vi "6733_Write_daqmx_87Sr.vi"(0 "Arbitrary Waveform\nArray of Channels":T1(array[cluster])=[[{"AC Frequency (kHz)"=40.0, " Initial AC Ampl. (p-p/2)"=0.0, "Final AC Ampl."=0.0, "Initial DC Value"=1.2, "Final DC Value"=0.6, "Constant"=80.29, "Gamma AC"=1.0, "String"="Channel 0 A", "Gamma DC"=1.0}, {"AC Frequency (kHz)"=40.0, " Initial AC Ampl. (p-p/2)"=0.0, "Final AC Ampl."=0.0, "Initial DC Value"=0.6, "Final DC Value"=0.2, "Constant"=80.29, "Gamma AC"=1.0, "String"="Channel 0 B", "Gamma DC"=1.0}, {"AC Frequency (kHz)"=40.0, " Initial AC Ampl. (p-p/2)"=0.0, "Final AC Ampl."=0.0, "Initial DC Value"=0.2, "Final DC Value"=0.075, "Constant"=80.29, "Gamma AC"=1.0, "String"="Channel 0 C", "Gamma DC"=1.0}, {"AC Frequency (kHz)"=0.0, " Initial AC Ampl. (p-p/2)"=0.0, "Final AC Ampl."=0.0, "Initial DC Value"=0.0, "Final DC Value"=1.8, "Constant"=84.5, "Gamma AC"=0.0, "String"="Channel 0 D", "Gamma DC"=1.0}, {"AC Frequency (kHz)"=0.0, " Initial AC Ampl. (p-p/2)"=0.0, "Final AC Ampl."=0.0, "Initial DC Value"=0.0, "Final DC Value"=0.0, "Constant"=81.22, "Gamma AC"=0.0, "String"="Channel 0 E", "Gamma DC"=1.0}, {"AC Frequency (kHz)"=0.0, " Initial AC Ampl. (p-p/2)"=0.0, "Final AC Ampl."=0.0, "Initial DC Value"=0.0, "Final DC Value"=0.0, "Constant"=86.0, "Gamma AC"=0.0, "String"="Channel 0 F", "Gamma DC"=1.0}], [{"AC Frequency (kHz)"=10.0, " Initial AC Ampl. (p-p/2)"=5.0, "Final AC Ampl."=0.0, "Initial DC Value"=1.0, "Final DC Value"=0.3, "Constant"=0.0, "Gamma AC"=1.0, "String"="Channel 1 A", "Gamma DC"=1.0}, {"AC Frequency (kHz)"=10.0, " Initial AC Ampl. (p-p/2)"=5.0, "Final AC Ampl."=0.0, "Initial DC Value"=0.3, "Final DC Value"=-0.8, "Constant"=0.0, "Gamma AC"=1.0, "String"="Channel 1 B", "Gamma DC"=1.0}, {"AC Frequency (kHz)"=10.0, " Initial AC Ampl. (p-p/2)"=0.0, "Final AC Ampl."=0.0, "Initial DC Value"=-0.8, "Final DC Value"=-0.8, "Constant"=0.0, "Gamma AC"=1.0, "String"="Channel 1 C", "Gamma DC"=1.0}, {"AC Frequency (kHz)"=0.0, " Initial AC Ampl. (p-p/2)"=0.0, "Final AC Ampl."=0.0, "Initial DC Value"=-1.0, "Final DC Value"=-1.0, "Constant"=0.0, "Gamma AC"=0.0, "String"="Channel 1 D", "Gamma DC"=1.0}, {"AC Frequency (kHz)"=0.0, " Initial AC Ampl. (p-p/2)"=0.0, "Final AC Ampl."=0.0, "Initial DC Value"=-1.0, "Final DC Value"=-1.0, "Constant"=0.0, "Gamma AC"=0.0, "String"="Channel 1E", "Gamma DC"=1.0}, {"AC Frequency (kHz)"=0.0, " Initial AC Ampl. (p-p/2)"=0.0, "Final AC Ampl."=0.0, "Initial DC Value"=-1.0, "Final DC Value"=-1.0, "Constant"=0.0, "Gamma AC"=0.0, "String"="", "Gamma DC"=1.0}], [{"AC Frequency (kHz)"=10.0, " Initial AC Ampl. (p-p/2)"=0.0, "Final AC Ampl."=0.0, "Initial DC Value"=0.01, "Final DC Value"=0.04, "Constant"=0.0, "Gamma AC"=1.0, "String"="Channel 2 A", "Gamma DC"=1.0}, {"AC Frequency (kHz)"=10.0, " Initial AC Ampl. (p-p/2)"=0.0, "Final AC Ampl."=0.0, "Initial DC Value"=0.04, "Final DC Value"=0.1, "Constant"=0.0, "Gamma AC"=1.0, "String"="Channel 2 B", "Gamma DC"=1.0}, {"AC Frequency (kHz)"=10.0, " Initial AC Ampl. (p-p/2)"=0.0, "Final AC Ampl."=0.0, "Initial DC Value"=0.1, "Final DC Value"=0.1, "Constant"=0.0, "Gamma AC"=1.0, "String"="Channel 2 C", "Gamma DC"=1.0}, {"AC Frequency (kHz)"=0.0, " Initial AC Ampl. (p-p/2)"=0.0, "Final AC Ampl."=0.0, "Initial DC Value"=0.1, "Final DC Value"=0.1, "Constant"=0.0, "Gamma AC"=0.0, "String"="Channel 2 D", "Gamma DC"=1.0}, {"AC Frequency (kHz)"=0.0, " Initial AC Ampl. (p-p/2)"=0.0, "Final AC Ampl."=0.0, "Initial DC Value"=0.1, "Final DC Value"=0.1, "Constant"=0.0, "Gamma AC"=0.0, "String"="", "Gamma DC"=1.0}, {"AC Frequency (kHz)"=0.0, " Initial AC Ampl. (p-p/2)"=0.0, "Final AC Ampl."=0.0, "Initial DC Value"=0.1, "Final DC Value"=0.1, "Constant"=0.0, "Gamma AC"=0.0, "String"="", "Gamma DC"=1.0}], [{"AC Frequency (kHz)"=10.0, " Initial AC Ampl. (p-p/2)"=0.0, "Final AC Ampl."=0.0, "Initial DC Value"=10.0, "Final DC Value"=10.0, "Constant"=199.25, "Gamma AC"=1.0, "String"="Channel 3 A", "Gamma DC"=1.0}, {"AC Frequency (kHz)"=10.0, " Initial AC Ampl. (p-p/2)"=0.0, "Final AC Ampl."=0.0, "Initial DC Value"=10.0, "Final DC Value"=0.8, "Constant"=199.25, "Gamma AC"=1.0, "String"="Channel 3 B", "Gamma DC"=1.0}, {"AC Frequency (kHz)"=10.0, " Initial AC Ampl. (p-p/2)"=0.0, "Final AC Ampl."=0.0, "Initial DC Value"=1.0, "Final DC Value"=0.5, "Constant"=199.25, "Gamma AC"=1.0, "String"="Channel 3 C", "Gamma DC"=1.0}, {"AC Frequency (kHz)"=0.0, " Initial AC Ampl. (p-p/2)"=0.0, "Final AC Ampl."=0.0, "Initial DC Value"=1.0, "Final DC Value"=1.0, "Constant"=199.25, "Gamma AC"=0.0, "String"="Channel 3 D", "Gamma DC"=1.0}, {"AC Frequency (kHz)"=0.0, " Initial AC Ampl. (p-p/2)"=0.0, "Final AC Ampl."=0.0, "Initial DC Value"=0.6, "Final DC Value"=0.6, "Constant"=199.2, "Gamma AC"=0.0, "String"="", "Gamma DC"=1.0}, {"AC Frequency (kHz)"=0.0, " Initial AC Ampl. (p-p/2)"=0.0, "Final AC Ampl."=0.0, "Initial DC Value"=0.6, "Final DC Value"=0.6, "Constant"=199.2, "Gamma AC"=0.0, "String"="", "Gamma DC"=1.0}], [{"AC Frequency (kHz)"=10.0, " Initial AC Ampl. (p-p/2)"=0.0, "Final AC Ampl."=0.0, "Initial DC Value"=-1.2, "Final DC Value"=-0.6, "Constant"=221.72, "Gamma AC"=1.0, "String"="Channel 4 A", "Gamma DC"=1.0}, {"AC Frequency (kHz)"=10.0, " Initial AC Ampl. (p-p/2)"=0.0, "Final AC Ampl."=0.0, "Initial DC Value"=-0.6, "Final DC Value"=-0.2, "Constant"=221.72, "Gamma AC"=1.0, "String"="Channel 4 B", "Gamma DC"=1.0}, {"AC Frequency (kHz)"=10.0, " Initial AC Ampl. (p-p/2)"=0.0, "Final AC Ampl."=0.0, "Initial DC Value"=-0.2, "Final DC Value"=-0.075, "Constant"=221.72, "Gamma AC"=1.0, "String"="Channel 4 C", "Gamma DC"=1.0}, {"AC Frequency (kHz)"=0.0, " Initial AC Ampl. (p-p/2)"=0.0, "Final AC Ampl."=0.0, "Initial DC Value"=0.0, "Final DC Value"=0.0, "Constant"=221.69, "Gamma AC"=0.0, "String"="Channel 4 D", "Gamma DC"=1.0}, {"AC Frequency (kHz)"=0.0, " Initial AC Ampl. (p-p/2)"=0.0, "Final AC Ampl."=0.0, "Initial DC Value"=0.0, "Final DC Value"=0.0, "Constant"=221.85, "Gamma AC"=0.0, "String"="", "Gamma DC"=1.0}, {"AC Frequency (kHz)"=0.0, " Initial AC Ampl. (p-p/2)"=0.0, "Final AC Ampl."=0.0, "Initial DC Value"=0.0, "Final DC Value"=0.0, "Constant"=221.85, "Gamma AC"=0.0, "String"="", "Gamma DC"=1.0}], [{"AC Frequency (kHz)"=10.0, " Initial AC Ampl. (p-p/2)"=0.0, "Final AC Ampl."=0.0, "Initial DC Value"=10.0, "Final DC Value"=10.0, "Constant"=0.0, "Gamma AC"=1.0, "String"="Channel 5 A", "Gamma DC"=1.0}, {"AC Frequency (kHz)"=10.0, " Initial AC Ampl. (p-p/2)"=0.0, "Final AC Ampl."=0.0, "Initial DC Value"=10.0, "Final DC Value"=0.8, "Constant"=0.0, "Gamma AC"=1.0, "String"="Channel 5 B", "Gamma DC"=1.0}, {"AC Frequency (kHz)"=10.0, " Initial AC Ampl. (p-p/2)"=0.0, "Final AC Ampl."=0.0, "Initial DC Value"=1.0, "Final DC Value"=0.5, "Constant"=0.0, "Gamma AC"=1.0, "String"="Channel 5 C", "Gamma DC"=1.0}, {"AC Frequency (kHz)"=0.0, " Initial AC Ampl. (p-p/2)"=0.0, "Final AC Ampl."=0.0, "Initial DC Value"=0.47, "Final DC Value"=0.47, "Constant"=0.0, "Gamma AC"=0.0, "String"="Channel 5 D", "Gamma DC"=1.0}, {"AC Frequency (kHz)"=0.0, " Initial AC Ampl. (p-p/2)"=0.0, "Final AC Ampl."=0.0, "Initial DC Value"=10.0, "Final DC Value"=10.0, "Constant"=0.0, "Gamma AC"=0.0, "String"="", "Gamma DC"=1.0}, {"AC Frequency (kHz)"=0.0, " Initial AC Ampl. (p-p/2)"=0.0, "Final AC Ampl."=0.0, "Initial DC Value"=10.0, "Final DC Value"=10.0, "Constant"=0.0, "Gamma AC"=0.0, "String"="", "Gamma DC"=1.0}], [{"AC Frequency (kHz)"=10.0, " Initial AC Ampl. (p-p/2)"=0.0, "Final AC Ampl."=0.0, "Initial DC Value"=1.0, "Final DC Value"=0.0, "Constant"=0.0, "Gamma AC"=1.0, "String"="Channel 6 A", "Gamma DC"=1.0}, {"AC Frequency (kHz)"=10.0, " Initial AC Ampl. (p-p/2)"=0.0, "Final AC Ampl."=0.0, "Initial DC Value"=0.0, "Final DC Value"=-0.7, "Constant"=0.0, "Gamma AC"=1.0, "String"="Channel 6 B", "Gamma DC"=1.0}, {"AC Frequency (kHz)"=10.0, " Initial AC Ampl. (p-p/2)"=0.0, "Final AC Ampl."=0.0, "Initial DC Value"=-0.8, "Final DC Value"=-0.8, "Constant"=0.0, "Gamma AC"=1.0, "String"="Channel 6 C", "Gamma DC"=1.0}, {"AC Frequency (kHz)"=0.0, " Initial AC Ampl. (p-p/2)"=0.0, "Final AC Ampl."=0.0, "Initial DC Value"=-1.0, "Final DC Value"=-1.0, "Constant"=0.0, "Gamma AC"=0.0, "String"="Channel 6 D", "Gamma DC"=1.0}, {"AC Frequency (kHz)"=0.0, " Initial AC Ampl. (p-p/2)"=0.0, "Final AC Ampl."=0.0, "Initial DC Value"=1.0, "Final DC Value"=1.0, "Constant"=0.0, "Gamma AC"=0.0, "String"="", "Gamma DC"=1.0}, {"AC Frequency (kHz)"=0.0, " Initial AC Ampl. (p-p/2)"=0.0, "Final AC Ampl."=0.0, "Initial DC Value"=1.0, "Final DC Value"=1.0, "Constant"=0.0, "Gamma AC"=0.0, "String"="", "Gamma DC"=1.0}], [{"AC Frequency (kHz)"=10.0, " Initial AC Ampl. (p-p/2)"=0.0, "Final AC Ampl."=0.0, "Initial DC Value"=1.0, "Final DC Value"=1.0, "Constant"=0.0, "Gamma AC"=1.0, "String"="Channel 7 A", "Gamma DC"=1.0}, {"AC Frequency (kHz)"=10.0, " Initial AC Ampl. (p-p/2)"=0.0, "Final AC Ampl."=0.0, "Initial DC Value"=1.0, "Final DC Value"=1.0, "Constant"=0.0, "Gamma AC"=1.0, "String"="Channel 7 B", "Gamma DC"=1.0}, {"AC Frequency (kHz)"=10.0, " Initial AC Ampl. (p-p/2)"=0.0, "Final AC Ampl."=0.0, "Initial DC Value"=1.0, "Final DC Value"=1.0, "Constant"=0.0, "Gamma AC"=1.0, "String"="Channel 7 C", "Gamma DC"=1.0}, {"AC Frequency (kHz)"=0.0, " Initial AC Ampl. (p-p/2)"=0.0, "Final AC Ampl."=0.0, "Initial DC Value"=1.0, "Final DC Value"=1.0, "Constant"=0.0, "Gamma AC"=0.0, "String"="Channel 7 D", "Gamma DC"=1.0}, {"AC Frequency (kHz)"=0.0, " Initial AC Ampl. (p-p/2)"=0.0, "Final AC Ampl."=0.0, "Initial DC Value"=1.0, "Final DC Value"=1.0, "Constant"=0.0, "Gamma AC"=0.0, "String"="", "Gamma DC"=1.0}, {"AC Frequency (kHz)"=0.0, " Initial AC Ampl. (p-p/2)"=0.0, "Final AC Ampl."=0.0, "Initial DC Value"=2.46, "Final DC Value"=2.46, "Constant"=199.2, "Gamma AC"=0.0, "String"="", "Gamma DC"=1.0}]] {"Gamma DC" format="%.2f"; "Gamma AC" format="%.2f"; "Constant" min=0.0 max=1250.0 format="%.2f"; "Final DC Value" format="%.3f"; "Initial DC Value" format="%.3f"; "Final AC Ampl." format="%.3f"; "Initial AC Ampl. (p-p/2)" format="%.3f"; "AC Frequency (kHz)" format="%.2f"}, 3 "Unit Conversions":u16[](array[ring])=[0, 2, 2, 3, 4, 3, 2, 2] items=["Freq (MHz) to Voltage 87Sr Trap", "87Sr Trap Dither Amplitude", "B-field to Voltage", "Power Control V for 689 nm (%)", "Freq (MHz) to Voltage 87Sr Stir", "Current (A) to Voltage Fet switch X trim", "87Sr Stir Dither Amplitude"], 4 "Interval Lengths (ms)":dbl[](array[numeric])=[200.0, 200.0, 100.0, 150.0, 1.0, 50.0] format="%.3f", 5 "Channel Controls":bool[](array[boolean])=[TRUE, TRUE, TRUE, TRUE, TRUE, TRUE, TRUE, TRUE], 6 "ON or OFF?":bool[](array[boolean])=[TRUE, TRUE, TRUE, TRUE, TRUE, TRUE], 7 "Hold Final Value of Array?":bool=TRUE, 9 "error in":errorcluster, 12 "Dither Control":u16(ring)=1 items=["Disable Dither", "Enable Dither"]) -> (8 "Voltage\nArrays":dbl[][](graph), 10 "= Total Waveform\nTime (ms)":dbl=651.0 format="%.3f", 11 "Sampling\nRate":dbl=3135.593220338983 format="%.2f", 14 "87Sr Trap V":dbl=2.8350019729729716, 15 "error out":errorcluster)   [LabVIEW 2013]
uses:
  <vilib>/Utility/error.llb/DialogType.ctl
  <vilib>/DAQmx/write.llb/DAQmx Write (Analog 1D Wfm NChan NSamp).vi
  <vilib>/DAQmx/configure/timing.llb/DAQmx Timing (Sample Clock).vi
  <vilib>/DAQmx/create/channels.llb/DAQmx Create Channel (CO-Pulse Generation-Frequency).vi
  <vilib>/DAQmx/configure/timing.llb/DAQmx Timing (Implicit).vi
  <vilib>/DAQmx/configure/trigger.llb/DAQmx Start Trigger (Digital Edge).vi
  Instance          13 29Saved   6733_Write_daqmx_87Sr .vi
  <vilib>/DAQmx/miscellaneous.llb/DAQmx Fill In Error Info.vi
  <resource>/objmgr/daqmx.rc
panel:
  in  "Case Constant\n(See Context Help) 3":bool=TRUE
  in  "Dither Control":u16
  in  "Dither Control":u16
  in  "Case Constant\n(See Context Help) 2":bool
  in  "Dither Control":u16
  in  "Case Constant\n(See Context Help)":bool
  in  "Dither Control":u16
  out "87Sr Stir V":dbl=5.786668445945946
  out "wvfrm size":i32=2040
  out "signal out":waveform(dbl)[](graph)=[{"t0"=timestamp(0 s since 1904-01-01), "dt"=0.00031891891891891894, "Y"=array[2040 elements]}, {"t0"=timestamp(0 s since 1904-01-01), "dt"=0.00031891891891891894, "Y"=array[2040 elements]}, {"t0"=timestamp(0 s since 1904-01-01), "dt"=0.00031891891891891894, "Y"=array[2040 elements]}, {"t0"=timestamp(0 s since 1904-01-01), "dt"=0.00031891891891891894, "Y"=array[2040 elements]}, {"t0"=timestamp(0 s since 1904-01-01), "dt"=0.00031891891891891894, "Y"=array[2040 elements]}, {"t0"=timestamp(0 s since 1904-01-01), "dt"=0.00031891891891891894, "Y"=array[2040 elements]}, {"t0"=timestamp(0 s since 1904-01-01), "dt"=0.00031891891891891894, "Y"=array[2040 elements]}, {"t0"=timestamp(0 s since 1904-01-01), "dt"=0.00031891891891891894, "Y"=array[2040 elements]}]
  out "87Sr 6733 counter task out":refnum<k21>="87Sr 6733 Counter Output"
  out "87Sr 6733 adiabatic loading task out":refnum<k21>="87Sr Red Waveform"
  out "6733 Status":string="PCI-6733 OK"
  out "total points\nper channel":dbl=2041.0 format="%.2f"
  out "Points per Segment":dbl[](array[numeric])=[627.0, 627.0, 313.0, 470.0, 3.0] format="%.2f"
  # "Controls"
  # "Warning! Constant for interval A does not set all intervals for 86 Sr frequency"
  # "Don't change"
  # "Note: B-field to Voltage\nConversion not yet\nimplemented.  Must \ninsert appropriate\nformulae."
  # "Interval A"
  # "Interval B"
  # "Interval C"
  # "Interval D"
  # "Interval E"
  # "Output"
  # "Must use all channels"
  # "CH 0"
  # "CH 1"
  # "CH 2"
  # "CH 3"
  # "CH 4"
  # "CH 5"
  # "CH 6"
  # "CH 7"
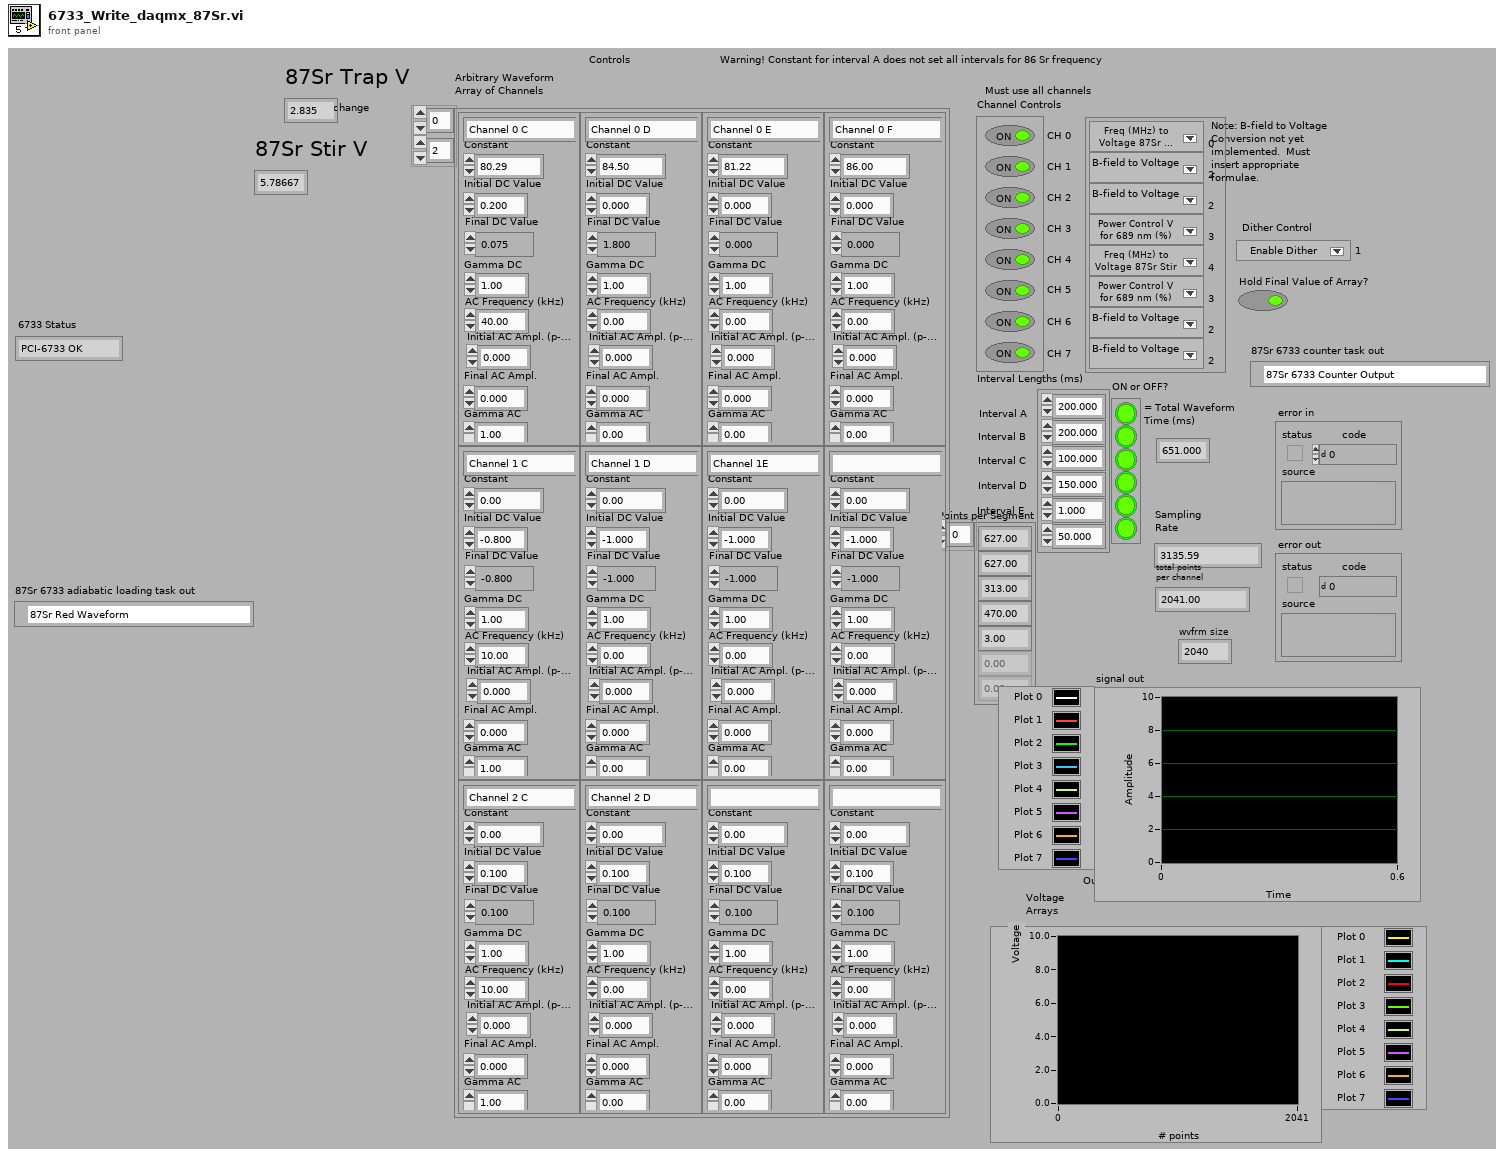
[diagram p1: front panel]
types:
  T1 = cluster{"AC Frequency (kHz)":dbl, " Initial AC Ampl. (p-p/2)":dbl, "Final AC Ampl.":dbl, "Initial DC Value":dbl, "Final DC Value":dbl, "Constant":dbl, "Gamma AC":dbl, "String":string, "Gamma DC":dbl}[][]
  T2 = cluster{"AC Frequency (kHz)":dbl, " Initial AC Ampl. (p-p/2)":dbl, "Final AC Ampl.":dbl, "Initial DC Value":dbl, "Final DC Value":dbl, "Constant":dbl, "Gamma AC":dbl, "String":string, "Gamma DC":dbl}
  T3 = typedef "DialogType.ctl" = u16
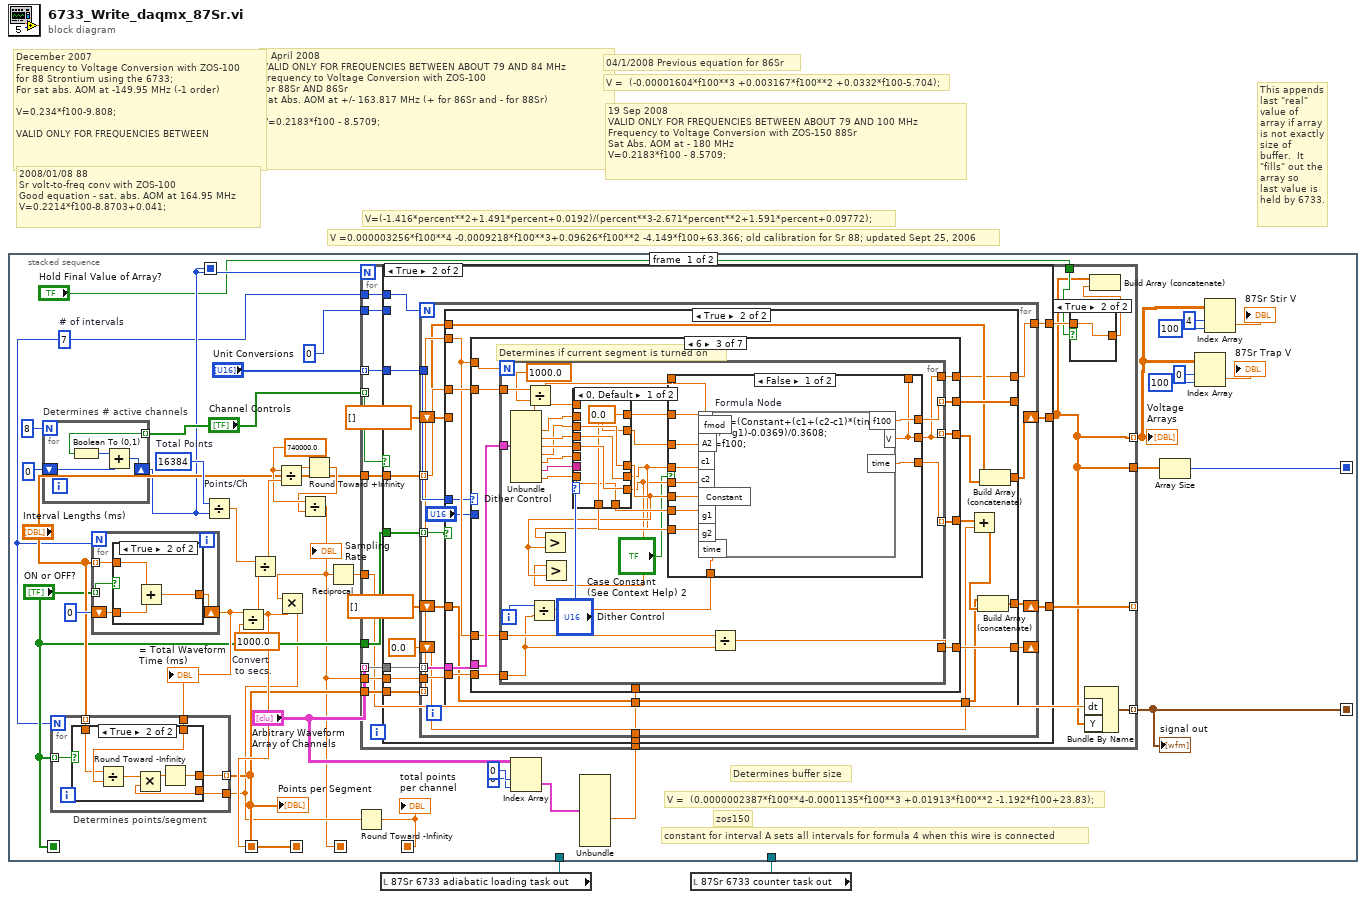
[diagram p0: block diagram]
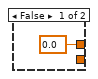
[diagram p2: hidden frame]
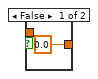
[diagram p4: hidden frame]
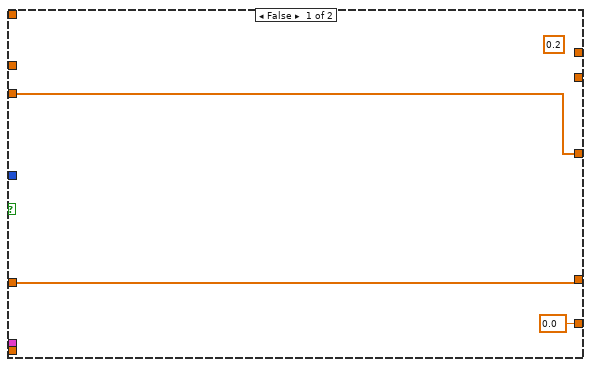
[diagram p6: hidden frame]
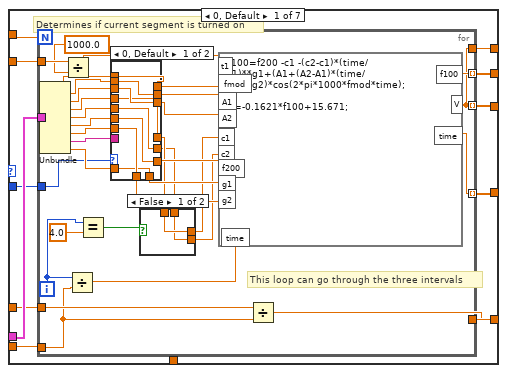
[diagram p7: hidden frame]
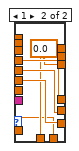
[diagram p9: hidden frame]
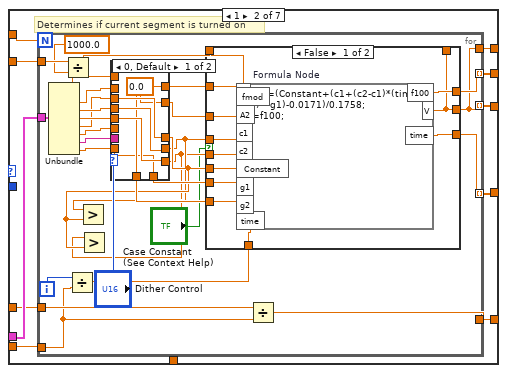
[diagram p10: hidden frame]
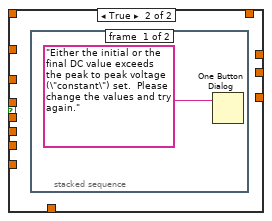
[diagram p11: hidden frame]
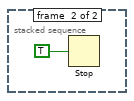
[diagram p12: hidden frame]
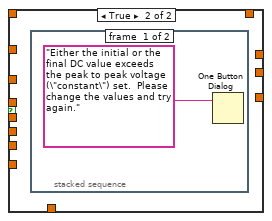
[diagram p14: hidden frame]
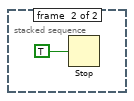
[diagram p15: hidden frame]
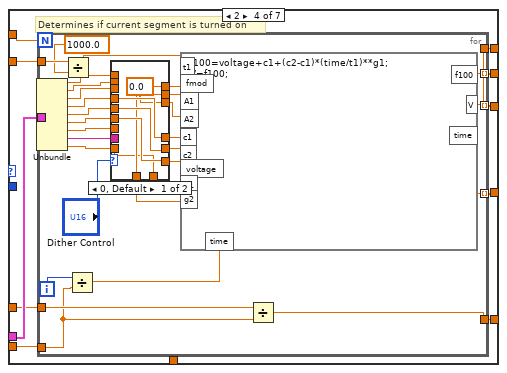
[diagram p17: hidden frame]
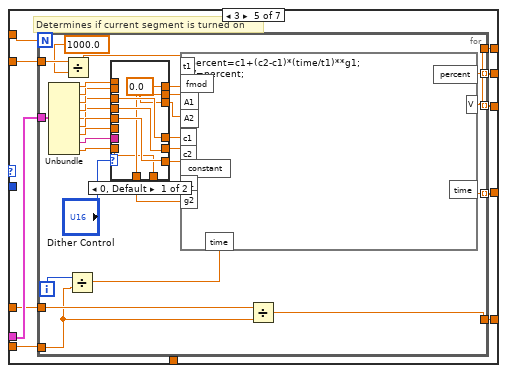
[diagram p19: hidden frame]
diagram:
  # "19 Sep 2008\nVALID ONLY FOR FREQUENCIES BETWEEN ABOUT 79 AND 100 MHz\nFrequency to Voltage Conversion with ZOS-150 88Sr\nSat Abs. AOM at - 180 MHz\nV=0.2183*f100 - 8.5709;"
  # "7 April 2008\nVALID ONLY FOR FREQUENCIES BETWEEN ABOUT 79 AND 84 MHz\nFrequency to Voltage Conversion with ZOS-100\nfor 88Sr AND 86Sr\nSat Abs. AOM at +/- 163.817 MHz (+ for 86Sr and - for 88Sr)\n\nV=0.2183*f100 - 8.5709;"
  # "04/1/2008 Previous equation for 86Sr"
  # "V =  (-0.00001604*f100**3 +0.003167*f100**2 +0.0332*f100-5.704);"
  # "December 2007\nFrequency to Voltage Conversion with ZOS-100\nfor 88 Strontium using the 6733; \nFor sat abs. AOM at -149.95 MHz (-1 order)\n\nV=0.234*f100-9.808;\n\nVALID ONLY FOR FREQUENCIES BETWEEN"
  # "2008/01/08 88\nSr volt-to-freq conv with ZOS-100\nGood equation - sat. abs. AOM at 164.95 MHz\nV=0.2214*f100-8.8703+0.041;"
  # "This appends\nlast \"real\"\nvalue of\narray if array \nis not exactly\nsize of \nbuffer.  It\n\"fills\" out the\narray so \nlast value is\nheld by 6733."
  # "V =0.000003256*f100**4 -0.0009218*f100**3+0.09626*f100**2 -4.149*f100+63.366; old calibration for Sr 88; updated Sept 25, 2006"
  # "V=(-1.416*percent**2+1.491*percent+0.0192)/(percent**3-2.671*percent**2+1.591*percent+0.09772);"
  n1 = local read "87Sr 6733 adiabatic loading task out"() -> (w2:refnum<k21>)
  n2 = local read "87Sr 6733 counter task out"() -> (w1:refnum<k21>)
  n3 = stacked-sequence {
    seq-local: [w13 _] -> [_ w543]
    seq-local: [w26 _] -> [_ _]
    seq-local: ["ON or OFF?" _] -> [_ _]
    seq-local: [w23 _] -> [_ _]
    seq-local: [w28 _] -> [_ _]
    seq-local: [w17 _] -> [_ w590]
    seq-local: [w14 _] -> [_ w542]
    seq-local: [w11 _] -> [_ w541]
    tunnel: w2 -> [_ w581]
    tunnel: w1 -> [_ w580]
    frame #0 {
      w32 = 740000.0 ("x")
      w10 = 7  # # of intervals
      w42 = 16384  # Total Points
      # "zos150"
      # "Determines buffer size"
      # "constant for interval A sets all intervals for formula 4 when this wire is connected"
      # "V =  (0.0000002387*f100**4-0.0001135*f100**3 +0.01913*f100**2 -1.192*f100+23.83);"
      n4 = for "Determines # active channels" {
        N: 8 -> [_]
        tunnel: "Channel Controls" -> [w66] mode=indexing
        shift-right: [w63] -> w17
        shift-left: 0 -> [w64]
        n5 = Boolean To (0,1)(Boolean=w66) -> (0, 1=w65:i16)
        n6 = Add(x=w65, y=w64) -> (x+y=w63:i32)
      }
      n7 = for {
        N: w10 -> [_]
        tunnel: "Interval Lengths (ms)" -> [w56] mode=indexing
        tunnel: "ON or OFF?" -> [w58] mode=indexing
        shift-right: [w55] -> w29
        shift-left: 0 -> [w57]
        n8 = case shown="True" w58 {
          tunnel: w57 -> [w59 w62]
          tunnel: w56 -> [_ w61]
          tunnel: [w59 w60] -> w55
          frame False {
          }
          frame True {
            n9 = Add(x=w61, y=w62) -> (x+y=w60:dbl)
          }
        }
      }
      "= Total Waveform\nTime (ms)" <- w29
      n10 = Divide "Points/Ch"(x=w42, y=w17) -> (x/y=w27:dbl)
      n11 = Divide "Convert\n to secs."(x=w29, y=1000.0) -> (x/y=w28:dbl)
      n12 = Divide(x=w27, y=w28) -> (x/y=w34:dbl)
      n13 = Divide(x=w32, y=w34) -> (x/y=w33:dbl)
      n14 = Round Toward +Infinity(x=w33) -> (ceil(x): smallest int >= x=w31:dbl)
      n15 = Divide(x=w32, y=w31) -> (x/y=w13:dbl)
      "Sampling\nRate" <- w13
      n16 = Multiply(x=w13, y=w28) -> (x*y=w24:dbl)
      n17 = for "Determines points/segment" {
        N: w10 -> [_]
        tunnel: "ON or OFF?" -> [w47] mode=indexing
        tunnel: "Interval Lengths (ms)" -> [w46] mode=indexing
        tunnel: w29 -> [w45]
        tunnel: [w44] -> w26 mode=indexing
        tunnel: w24 -> [w43]
        n18 = case shown="True" w47 {
          tunnel: w46 -> [_ w53]
          tunnel: w45 -> [_ w54]
          tunnel: [0.0 w50] -> w44
          tunnel: w43 -> [_ w51]
          frame False {
          }
          frame True {
            n19 = Divide(x=w53, y=w54) -> (x/y=w52:dbl)
            n20 = Multiply(x=w52, y=w51) -> (x*y=w49:dbl)
            n21 = Round Toward -Infinity(1:w49) -> (0:w50:dbl)
          }
        }
      }
      "Points per Segment" <- w26
      n22 = Reciprocal(x=w13) -> (1/x=w15:dbl)
      n23 = Round Toward -Infinity(1:w24) -> (0:w23:dbl)
      "total points\nper channel" <- w23
      n24 = Index Array(array="Arbitrary Waveform\nArray of Channels", index (row)=0, index (col)=0 ("disabled index (col)")) -> (element=w19:T2)
      n25 = Unbundle(w19) -> ("Constant"=w18:dbl)  [unwired: 8 out]
      n26 = for {
        N: w17 -> [_]
        tunnel: "Channel Controls" -> [w83] mode=indexing
        tunnel: 0 -> [w82]
        tunnel: "Unit Conversions" -> [w80] mode=indexing
        tunnel: "Arbitrary Waveform\nArray of Channels" -> [w81] mode=indexing
        tunnel: w26 -> [w79]
        tunnel: w13 -> [w70]
        tunnel: "Interval Lengths (ms)" -> [w78]
        tunnel: "ON or OFF?" -> [w77]
        tunnel: [w76] -> _ mode=indexing
        tunnel: [w67] -> w3 mode=indexing
        tunnel: w18 -> [w75]
        tunnel: "Hold Final Value of Array?" -> [w72]
        tunnel: [w71] -> w14 mode=indexing
        tunnel: w15 -> [w69]
        tunnel: [w67] -> w12
        tunnel: w10 -> [w68]
        n27 = case shown="True" w83 {
          tunnel: w82 -> [_ _]
          tunnel: w81 -> [_ w99]
          tunnel: w80 -> [_ w98]
          tunnel: w79 -> [_ w97]
          tunnel: w70 -> [_ w96]
          tunnel: w78 -> [_ w95]
          tunnel: w77 -> [_ w94]
          tunnel: [_ w92] -> w76
          tunnel: [_ w87] -> w67
          tunnel: w75 -> [_ w89]
          tunnel: [_ w86] -> w74
          tunnel: w68 -> [_ w88]
          frame False {
          }
          frame True {
            n28 = for {
              N: w88 -> [_]
              tunnel: w99 -> [w111] mode=indexing
              tunnel: w98 -> [w113]
              tunnel: w97 -> [w112] mode=indexing
              tunnel: w96 -> [w110]
              tunnel: w95 -> [w109] mode=indexing
              tunnel: w94 -> [w108] mode=indexing
              shift-right: [w107] -> w92
              shift-left: dbl[] [] -> [w106]
              shift-right: [w105] -> _
              shift-left: 0.0 -> [w104]
              shift-right: [w101] -> w87
              shift-left: dbl[] [] -> [w103]
              tunnel: w89 -> [w102]
              tunnel: [w100] -> w86
              n29 = case shown="True" w108 {
                tunnel: w113 -> [_ w120]
                tunnel: w112 -> [_ w126]
                tunnel: w111 -> [_ w134]
                tunnel: w110 -> [_ w133]
                tunnel: w109 -> [_ w132]
                tunnel: [_ w131] -> _
                tunnel: [w116 w130] -> w107
                tunnel: w106 -> [w116 w124]
                tunnel: [0.0 w128] -> w105
                tunnel: w104 -> [_ w127]
                tunnel: [w114 w123] -> w101
                tunnel: w103 -> [_ w121]
                tunnel: w103 -> [w114 _]
                tunnel: w102 -> [_ w118]
                tunnel: [_ w117] -> w100
                frame False {
                  (unwired) 0.2 ("V")
                }
                frame True {
                  n30 = case shown="6" w120 {
                    tunnel: w126 -> [w145 w205 w270 w335 w388 w443 w497]
                    tunnel: w134 -> [w144 w204 w269 w334 w387 w442 w496]
                    tunnel: w133 -> [w139 w199 w264 w329 w382 w437 w491]
                    tunnel: w132 -> [w143 w203 w268 w333 w386 w441 w495]
                    tunnel: [w142 w202 w267 w332 w385 w440 w494] -> w131
                    tunnel: [w141 w201 w266 w331 w384 w439 w493] -> w122
                    tunnel: [w140 w200 w265 w330 w383 w438 w492] -> w129
                    tunnel: [w138 w198 w263 w328 w381 w436 w490] -> w128
                    tunnel: w126 -> [w137 w197 w262 w327 w380 w435 w489]
                    tunnel: "Dither Control" -> [w136 _ _ _ _ w434 w488]
                    tunnel: w118 -> [_ _ _ _ _ w433 _]
                    tunnel: [w135 w196 w261 w326 w379 w432 w487] -> w117
                    frame 0, Default {
                      # "Determines if current segment is turned on"
                      n31 = for {
                        N: w145 -> [_]
                        tunnel: w144 -> [w179]
                        tunnel: w139 -> [w160]
                        tunnel: w143 -> [w178]
                        tunnel: [w146] -> w141 mode=indexing
                        tunnel: [w158] -> w140 mode=indexing
                        tunnel: [w157] -> w142 mode=indexing
                        tunnel: [w159] -> w138
                        tunnel: w137 -> [w161]
                        tunnel: w136 -> [w156]
                        tunnel: [w146] -> w135
                        i -> [w148]
                        # "EQUATION TO USE WITH SAT. ABS. AOM AT -180 MHz FOR 87SR TRAPPING LASER:\nV=-0.1621*f100+15.671"
                        # "This loop can go through the three intervals"
                        n32 = Unbundle(w179) -> ("AC Frequency (kHz)"=w173:dbl, "Initial AC Ampl. (p-p/2)"=w172:dbl, "Final AC Ampl."=w171:dbl, "Initial DC Value"=w155:dbl, "Final DC Value"=w170:dbl, "Constant"=w174:dbl, "Gamma AC"=w175:dbl, "String"=w176:string, "Gamma DC"=w164:dbl)
                        n33 = Divide(x=w178, y=1000.0) -> (x/y=w147:dbl)
                        n34 = Divide(x=w148, y=w160) -> (x/y=w162:dbl)
                        n35 = Equal?(x=w148, y=4.0) -> (x = y?=w153:bool)
                        n36 = case shown="0, Default" w156 {
                          tunnel: w176 -> [_ _]
                          tunnel: w175 -> [w184 _]
                          tunnel: w174 -> [w185 w193]
                          tunnel: w173 -> [w190 _]
                          tunnel: w172 -> [w189 _]
                          tunnel: w171 -> [w188 _]
                          tunnel: w155 -> [w187 w195]
                          tunnel: w170 -> [w186 w194]
                          tunnel: [w190 w192] -> w169
                          tunnel: [w189 w192] -> w168
                          tunnel: [w188 w192] -> w167
                          tunnel: [w187 w195] -> w152
                          tunnel: [w186 w194] -> w151
                          tunnel: [w185 w193] -> w166
                          tunnel: [w184 w192] -> w165
                          tunnel: w164 -> [w183 w191]
                          tunnel: [w183 w191] -> w163
                          frame 0, Default {
                          }
                          frame 1 {
                            w192 = 0.0 ("AC Frequency (kHz)")
                          }
                        }
                        n37 = case shown="False" w153 {
                          tunnel: [w181 w182] -> w150
                          tunnel: w152 -> [w181 w182]
                          tunnel: [w180 w182] -> w149
                          tunnel: w151 -> [w180 _]
                          frame False {
                          }
                          frame True {
                          }
                        }
                        n38 = formula code="f100=f200 -c1 -(c2-c1)*(time/t1)**g1+(A1+(A2-A1)*(time/t1)**g2)*cos(2*pi*1000*fmod*time);\n\nV=-0.1621*f100+15.671;"("c1"=w150, "time"=w162, "t1"=w147, "c2"=w149, "f200"=w166, "fmod"=w169, "A1"=w168, "A2"=w167, "g1"=w163, "g2"=w165) -> ("f100"=w157:dbl, "time"=w158:dbl, "V"=w146:dbl)
                        n39 = Divide(x=w161, y=w160) -> (x/y=w159:dbl)
                      }
                    }
                    frame 1 {
                      # "Determines if current segment is turned on"
                      n40 = for {
                        N: w205 -> [_]
                        tunnel: w204 -> [w234]
                        tunnel: w199 -> [w218]
                        tunnel: w203 -> [w231]
                        tunnel: [w207] -> w201 mode=indexing
                        tunnel: [w233] -> w200 mode=indexing
                        tunnel: [w232] -> w202 mode=indexing
                        tunnel: [w217] -> w198
                        tunnel: w197 -> [w219]
                        tunnel: [w207] -> w196
                        i -> [w229]
                        n41 = Unbundle(w234) -> ("AC Frequency (kHz)"=w211:dbl, "Final AC Ampl."=w212:dbl, "Initial DC Value"=w215:dbl, "Final DC Value"=w214:dbl, "Constant"=w213:dbl, "Gamma AC"=w227:dbl, "String"=w228:string, "Gamma DC"=w222:dbl)  [unwired: 1 out]
                        n42 = Divide(x=w231, y=1000.0) -> (x/y=w226:dbl)
                        n43 = Divide(x=w229, y=w218) -> (x/y=w220:dbl)
                        n44 = case shown="0, Default" "Dither Control" {
                          tunnel: w228 -> [_ _]
                          tunnel: w227 -> [_ w256]
                          tunnel: w214 -> [w251 w257]
                          tunnel: w212 -> [_ w260]
                          tunnel: w213 -> [w253 w259]
                          tunnel: w215 -> [w252 w258]
                          tunnel: [w250 w254] -> w225
                          tunnel: [w250 w260] -> w224
                          tunnel: [w253 w259] -> w210
                          tunnel: [w252 w258] -> w209
                          tunnel: [w251 w257] -> w208
                          tunnel: [w250 w256] -> w223
                          tunnel: w222 -> [w249 w255]
                          tunnel: [w249 w255] -> w221
                          tunnel: w211 -> [_ w254]
                          frame 0, Default {
                            w250 = 0.0 ("AC Frequency (kHz)")
                          }
                          frame 1 {
                          }
                        }
                        n45 = Greater?(x=w209, y=w210) -> ()  [unwired: 1 out]
                        n46 = Greater?(x=w208, y=w210) -> ()  [unwired: 1 out]
                        n47 = case shown="False" "Case Constant\n(See Context Help)" {
                          tunnel: [w235 _] -> w207
                          tunnel: [w246 _] -> w233
                          tunnel: [w245 _] -> w232
                          tunnel: w226 -> [w244 _]
                          tunnel: w225 -> [w243 _]
                          tunnel: w224 -> [w242 _]
                          tunnel: w223 -> [w241 _]
                          tunnel: w221 -> [w240 _]
                          tunnel: w220 -> [w239 _]
                          tunnel: w209 -> [w238 _]
                          tunnel: w208 -> [w237 _]
                          tunnel: w210 -> [w236 _]
                          tunnel: [w235 _] -> _
                          frame False {
                            # "Trap Dither amplitude control"
                            n48 = formula code="f100=(Constant+(c1+(c2-c1)*(time/t1)**g1)-0.0171)/0.1758;\nV=f100;"("c1"=w238, "time"=w239, "t1"=w244, "c2"=w237, "Constant"=w236, "fmod"=w243, "A2"=w242, "g1"=w240, "g2"=w241) -> ("f100"=w245:dbl, "time"=w246:dbl, "V"=w235:dbl)
                          }
                          frame True {
                            n49 = stacked-sequence {
                              frame #0 {
                                n50 = One Button Dialog(message="Either the initial or the final DC value exceeds the peak to peak voltage (\"constant\") set.  Please change the values and try again.") -> ()  [unwired: 1 in, 1 out]
                              }
                              frame #1 {
                                n51 = Stop(stop? (T)=TRUE) -> ()
                              }
                            }
                          }
                        }
                        n52 = Divide(x=w219, y=w218) -> (x/y=w217:dbl)
                      }
                    }
                    frame 6 {
                      # "Determines if current segment is turned on"
                      n53 = for {
                        N: w270 -> [_]
                        tunnel: w269 -> [w299]
                        tunnel: w264 -> [w283]
                        tunnel: w268 -> [w296]
                        tunnel: [w272] -> w266 mode=indexing
                        tunnel: [w298] -> w265 mode=indexing
                        tunnel: [w297] -> w267 mode=indexing
                        tunnel: [w282] -> w263
                        tunnel: w262 -> [w284]
                        tunnel: [w272] -> w261
                        i -> [w294]
                        n54 = Unbundle(w299) -> ("AC Frequency (kHz)"=w276:dbl, "Final AC Ampl."=w277:dbl, "Initial DC Value"=w280:dbl, "Final DC Value"=w279:dbl, "Constant"=w278:dbl, "Gamma AC"=w292:dbl, "String"=w293:string, "Gamma DC"=w287:dbl)  [unwired: 1 out]
                        n55 = Divide(x=w296, y=1000.0) -> (x/y=w291:dbl)
                        n56 = Divide(x=w294, y=w283) -> (x/y=w285:dbl)
                        n57 = case shown="0, Default" "Dither Control" {
                          tunnel: w293 -> [_ _]
                          tunnel: w292 -> [_ w321]
                          tunnel: w279 -> [w316 w322]
                          tunnel: w277 -> [_ w325]
                          tunnel: w278 -> [w318 w324]
                          tunnel: w280 -> [w317 w323]
                          tunnel: [w315 w319] -> w290
                          tunnel: [w315 w325] -> w289
                          tunnel: [w318 w324] -> w275
                          tunnel: [w317 w323] -> w274
                          tunnel: [w316 w322] -> w273
                          tunnel: [w315 w321] -> w288
                          tunnel: w287 -> [w314 w320]
                          tunnel: [w314 w320] -> w286
                          tunnel: w276 -> [_ w319]
                          frame 0, Default {
                            w315 = 0.0 ("AC Frequency (kHz)")
                          }
                          frame 1 {
                          }
                        }
                        n58 = Greater?(x=w274, y=w275) -> ()  [unwired: 1 out]
                        n59 = Greater?(x=w273, y=w275) -> ()  [unwired: 1 out]
                        n60 = case shown="False" "Case Constant\n(See Context Help) 2" {
                          tunnel: [w300 _] -> w272
                          tunnel: [w311 _] -> w298
                          tunnel: [w310 _] -> w297
                          tunnel: w291 -> [w309 _]
                          tunnel: w290 -> [w308 _]
                          tunnel: w289 -> [w307 _]
                          tunnel: w288 -> [w306 _]
                          tunnel: w286 -> [w305 _]
                          tunnel: w285 -> [w304 _]
                          tunnel: w274 -> [w303 _]
                          tunnel: w273 -> [w302 _]
                          tunnel: w275 -> [w301 _]
                          tunnel: [w300 _] -> _
                          frame False {
                            # "Stir Dither amplitude control"
                            n61 = formula code="f100=(Constant+(c1+(c2-c1)*(time/t1)**g1)-0.0369)/0.3608;\nV=f100;"("c1"=w303, "time"=w304, "t1"=w309, "c2"=w302, "Constant"=w301, "fmod"=w308, "A2"=w307, "g1"=w305, "g2"=w306) -> ("f100"=w310:dbl, "time"=w311:dbl, "V"=w300:dbl)
                          }
                          frame True {
                            n62 = stacked-sequence {
                              frame #0 {
                                n63 = One Button Dialog(message="Either the initial or the final DC value exceeds the peak to peak voltage (\"constant\") set.  Please change the values and try again.") -> ()  [unwired: 1 in, 1 out]
                              }
                              frame #1 {
                                n64 = Stop(stop? (T)=TRUE) -> ()
                              }
                            }
                          }
                        }
                        n65 = Divide(x=w284, y=w283) -> (x/y=w282:dbl)
                      }
                    }
                    frame 2 {
                      # "Determines if current segment is turned on"
                      n66 = for {
                        N: w335 -> [_]
                        tunnel: w334 -> [w365]
                        tunnel: w329 -> [w339]
                        tunnel: w333 -> [w362]
                        tunnel: [w336] -> w331 mode=indexing
                        tunnel: [w364] -> w330 mode=indexing
                        tunnel: [w363] -> w332 mode=indexing
                        tunnel: [w338] -> w328
                        tunnel: w327 -> [w340]
                        tunnel: [w336] -> w326
                        i -> [w360]
                        # "B-field to voltage"
                        n67 = Unbundle(w365) -> ("AC Frequency (kHz)"=w356:dbl, "Initial AC Ampl. (p-p/2)"=w355:dbl, "Final AC Ampl."=w354:dbl, "Initial DC Value"=w353:dbl, "Final DC Value"=w352:dbl, "Constant"=w357:dbl, "Gamma AC"=w358:dbl, "String"=w359:string, "Gamma DC"=w343:dbl)
                        n68 = Divide(x=w362, y=1000.0) -> (x/y=w351:dbl)
                        n69 = Divide(x=w360, y=w339) -> (x/y=w341:dbl)
                        n70 = case shown="0, Default" "Dither Control" {
                          tunnel: w359 -> [_ _]
                          tunnel: w358 -> [_ w372]
                          tunnel: w357 -> [w368 w373]
                          tunnel: w356 -> [_ w378]
                          tunnel: w355 -> [_ w377]
                          tunnel: w354 -> [_ w376]
                          tunnel: w353 -> [w370 w375]
                          tunnel: w352 -> [w369 w374]
                          tunnel: [w367 w378] -> w350
                          tunnel: [w367 w377] -> w349
                          tunnel: [w367 w376] -> w348
                          tunnel: [w370 w375] -> w347
                          tunnel: [w369 w374] -> w346
                          tunnel: [w368 w373] -> w345
                          tunnel: [w367 w372] -> w344
                          tunnel: w343 -> [w366 w371]
                          tunnel: [w366 w371] -> w342
                          frame 0, Default {
                            w367 = 0.0 ("AC Frequency (kHz)")
                          }
                          frame 1 {
                          }
                        }
                        n71 = formula code="f100=voltage+c1+(c2-c1)*(time/t1)**g1;\nV=f100;"("c1"=w347, "time"=w341, "t1"=w351, "c2"=w346, "voltage"=w345, "fmod"=w350, "A1"=w349, "A2"=w348, "g1"=w342, "g2"=w344) -> ("f100"=w363:dbl, "time"=w364:dbl, "V"=w336:dbl)
                        n72 = Divide(x=w340, y=w339) -> (x/y=w338:dbl)
                      }
                    }
                    frame 3 {
                      # "Determines if current segment is turned on"
                      n73 = for {
                        N: w388 -> [_]
                        tunnel: w387 -> [w418]
                        tunnel: w382 -> [w392]
                        tunnel: w386 -> [w415]
                        tunnel: [w389] -> w384 mode=indexing
                        tunnel: [w417] -> w383 mode=indexing
                        tunnel: [w416] -> w385 mode=indexing
                        tunnel: [w391] -> w381
                        tunnel: w380 -> [w393]
                        tunnel: [w389] -> w379
                        i -> [w413]
                        # "Power Control Voltage for 689 nm\npercent = 1 is full power"
                        n74 = Unbundle(w418) -> ("AC Frequency (kHz)"=w409:dbl, "Initial AC Ampl. (p-p/2)"=w408:dbl, "Final AC Ampl."=w407:dbl, "Initial DC Value"=w406:dbl, "Final DC Value"=w405:dbl, "Constant"=w410:dbl, "Gamma AC"=w411:dbl, "String"=w412:string, "Gamma DC"=w396:dbl)
                        n75 = Divide(x=w415, y=1000.0) -> (x/y=w404:dbl)
                        n76 = Divide(x=w413, y=w392) -> (x/y=w394:dbl)
                        n77 = case shown="0, Default" "Dither Control" {
                          tunnel: w412 -> [_ _]
                          tunnel: w411 -> [_ w425]
                          tunnel: w410 -> [w421 w426]
                          tunnel: w409 -> [_ w431]
                          tunnel: w408 -> [_ w430]
                          tunnel: w407 -> [_ w429]
                          tunnel: w406 -> [w423 w428]
                          tunnel: w405 -> [w422 w427]
                          tunnel: [w420 w431] -> w403
                          tunnel: [w420 w430] -> w402
                          tunnel: [w420 w429] -> w401
                          tunnel: [w423 w428] -> w400
                          tunnel: [w422 w427] -> w399
                          tunnel: [w421 w426] -> w398
                          tunnel: [w420 w425] -> w397
                          tunnel: w396 -> [w419 w424]
                          tunnel: [w419 w424] -> w395
                          frame 0, Default {
                            w420 = 0.0 ("AC Frequency (kHz)")
                          }
                          frame 1 {
                          }
                        }
                        n78 = formula code="percent=c1+(c2-c1)*(time/t1)**g1;\nV=percent;"("c1"=w400, "time"=w394, "t1"=w404, "c2"=w399, "constant"=w398, "fmod"=w403, "A1"=w402, "A2"=w401, "g1"=w395, "g2"=w397) -> ("percent"=w416:dbl, "time"=w417:dbl, "V"=w389:dbl)
                        n79 = Divide(x=w393, y=w392) -> (x/y=w391:dbl)
                      }
                    }
                    frame 4 {
                      # "Determines if current segment is turned on"
                      n80 = for {
                        N: w443 -> [_]
                        tunnel: w442 -> [w473]
                        tunnel: w437 -> [w450]
                        tunnel: w441 -> [w472]
                        tunnel: [w444] -> w439 mode=indexing
                        tunnel: [w448] -> w438 mode=indexing
                        tunnel: [w447] -> w440 mode=indexing
                        tunnel: [w449] -> w436
                        tunnel: w435 -> [w451]
                        tunnel: w434 -> [w446]
                        tunnel: w433 -> [_]
                        tunnel: [w445] -> _ mode=indexing
                        tunnel: [w444] -> w432
                        i -> [w470]
                        # "EQUATION TO USE WITH SAT. ABS. AOM AT -180 MHz FOR 87SR STIR LASER:\nV=-0.07955*f100+16.3155"
                        # "zos100"
                        # "constant"
                        n81 = Unbundle(w473) -> ("AC Frequency (kHz)"=w467:dbl, "Initial AC Ampl. (p-p/2)"=w466:dbl, "Final AC Ampl."=w465:dbl, "Initial DC Value"=w464:dbl, "Final DC Value"=w463:dbl, "Constant"=w445:dbl, "Gamma AC"=w468:dbl, "String"=w469:string, "Gamma DC"=w454:dbl)
                        n82 = Divide(x=w472, y=1000.0) -> (x/y=w462:dbl)
                        n83 = Divide(x=w470, y=w450) -> (x/y=w452:dbl)
                        n84 = case shown="0, Default" w446 {
                          tunnel: w469 -> [_ _]
                          tunnel: w468 -> [w475 _]
                          tunnel: w445 -> [w476 w484]
                          tunnel: w467 -> [w481 _]
                          tunnel: w466 -> [w480 _]
                          tunnel: w465 -> [w479 _]
                          tunnel: w464 -> [w478 w486]
                          tunnel: w463 -> [w477 w485]
                          tunnel: [w481 w483] -> w461
                          tunnel: [w480 w483] -> w460
                          tunnel: [w479 w483] -> w459
                          tunnel: [w478 w486] -> w458
                          tunnel: [w477 w485] -> w457
                          tunnel: [w476 w484] -> w456
                          tunnel: [w475 w483] -> w455
                          tunnel: w454 -> [w474 w482]
                          tunnel: [w474 w482] -> w453
                          frame 0, Default {
                          }
                          frame 1 {
                            w483 = 0.0 ("AC Frequency (kHz)")
                          }
                        }
                        n85 = formula code="f100=f200-90-c1 -(c2-c1)*(time/t1)**g1+(A1+(A2-A1)*(time/t1)**g2)*cos(2*pi*1000*fmod*time);\n\nV=-0.078915*f100+16.2685;"("c1"=w458, "time"=w452, "t1"=w462, "c2"=w457, "f200"=w456, "fmod"=w461, "A1"=w460, "A2"=w459, "g1"=w453, "g2"=w455) -> ("f100"=w447:dbl, "time"=w448:dbl, "V"=w444:dbl)
                        n86 = Divide(x=w451, y=w450) -> (x/y=w449:dbl)
                      }
                    }
                    frame 5 {
                      # "Determines if current segment is turned on"
                      n87 = for {
                        N: w497 -> [_]
                        tunnel: w496 -> [w527]
                        tunnel: w491 -> [w504]
                        tunnel: w495 -> [w526]
                        tunnel: [w498] -> w493 mode=indexing
                        tunnel: [w502] -> w492 mode=indexing
                        tunnel: [w501] -> w494 mode=indexing
                        tunnel: [w503] -> w490
                        tunnel: w489 -> [w505]
                        tunnel: w488 -> [w500]
                        tunnel: [w498] -> w487
                        i -> [w524]
                        # "Use V=c1 to be able to change c1 and c2\nprovided c1 and c2 match."
                        # "current to voltage conversion for FET\n switch  driving X trim coils. Derivation on\n Neutrals Notebook A pg 87 yellow"
                        # "This loop can go through the three intervals"
                        n88 = Unbundle(w527) -> ("AC Frequency (kHz)"=w520:dbl, "Initial AC Ampl. (p-p/2)"=w519:dbl, "Final AC Ampl."=w518:dbl, "Initial DC Value"=w499:dbl, "Final DC Value"=w517:dbl, "Constant"=w521:dbl, "Gamma AC"=w522:dbl, "String"=w523:string, "Gamma DC"=w508:dbl)
                        n89 = Divide(x=w526, y=1000.0) -> (x/y=w516:dbl)
                        n90 = Divide(x=w524, y=w504) -> (x/y=w506:dbl)
                        n91 = case shown="1" w500 {
                          tunnel: w523 -> [_ _]
                          tunnel: w522 -> [w529 _]
                          tunnel: w521 -> [w530 w538]
                          tunnel: w520 -> [w535 _]
                          tunnel: w519 -> [w534 _]
                          tunnel: w518 -> [w533 _]
                          tunnel: w499 -> [w532 w540]
                          tunnel: w517 -> [w531 w539]
                          tunnel: [w535 w537] -> w515
                          tunnel: [w534 w537] -> w514
                          tunnel: [w533 w537] -> w513
                          tunnel: [w532 w540] -> w512
                          tunnel: [w531 w539] -> w511
                          tunnel: [w530 w538] -> w510
                          tunnel: [w529 w537] -> w509
                          tunnel: w508 -> [w528 w536]
                          tunnel: [w528 w536] -> w507
                          frame 0, Default {
                          }
                          frame 1 {
                            w537 = 0.0 ("AC Frequency (kHz)")
                          }
                        }
                        n92 = formula code="f100=f200 +c1 +(c2-c1)*(time/t1)**g1;\n\nV=f100;"("c1"=w512, "time"=w506, "t1"=w516, "c2"=w511, "f200"=w510, "fmod"=w515, "A1"=w514, "A2"=w513, "g1"=w507, "g2"=w509) -> ("f100"=w501:dbl, "time"=w502:dbl, "V"=w498:dbl)
                        n93 = Divide(x=w505, y=w504) -> (x/y=w503:dbl)
                      }
                    }
                  }
                  n94 = Add(x=w129, y=w127) -> (x+y=w125:dbl[])
                  n95 = Build Array (concatenate)(w124, w125) -> (w130:dbl[])
                  n96 = Build Array (concatenate)(w121, w122) -> (w123:dbl[])
                }
              }
            }
          }
        }
        n97 = case shown="True" w72 {
          tunnel: [0.0 w85] -> w73
          tunnel: w74 -> [_ w85]
          frame False {
          }
          frame True {
          }
        }
        n98 = Bundle By Name("dt"=w69, "Y"=w67) -> (w71:waveform(dbl))  [unwired: 1 in]
        n99 = Build Array (concatenate)(w67, w73) -> ()  [unwired: 1 out]
      }
      "Voltage\nArrays" <- w3
      "signal out" <- w14
      n100 = Array Size(array=w12) -> (size(s)=w11:i32)
      n101 = Index Array(array=w3, index (row)=0, index (col)=100 ("disabled index (col)")) -> (element=→"87Sr Trap V":dbl)
      n102 = Index Array(array=w3, index (row)=4, index (col)=100 ("disabled index (col)")) -> (element=→"87Sr Stir V":dbl)
    }
    frame #1 {
      w544 = T3 3 items=["no dialog", "OK message", "continue or stop message", "OK message + warnings", "continue/stop + warnings"] ("type of dialog (OK msg:1)")
      w545 = 10123 items=["Finite Samples"=10178, "Continuous Samples"=10123, "Hardware Timed Single Point"=12522] ("sample mode")
      w546 = 10280 items=["Rising"=10280, "Falling"=10171] ("edge")
      w556 = 10214 items=["High"=10192, "Low"=10214] ("idle state")
      w557 = 10178 items=["Finite Samples"=10178, "Continuous Samples"=10123, "Hardware Timed Single Point"=12522] ("sample mode")
      # "Counter Channel"
      # "Physical Channel"
      # "device 1:\nnew 6733 board\ncheck NI MAX if in doubt"
      # "task ID is an output of this VI; it is used to close the 6733 later in the program.\nDo not delete!"
      # "sampling rate"
      # "total points per channel"
      # "Points per segment"
      # "write voltage values to intermediate buffer"
      # "write waveform"
      # "Configure counter\nfor retriggerable AO"
      n103 = case shown="8" w590 {
        tunnel: [_ refnum<k21> "87Sr 6733 AO 00" ("global virtual channels") refnum<k21> "87Sr 6733 AO 00:01" ("global virtual channels") refnum<k21> "87Sr 6733 AO 00:02" ("global virtual channels") refnum<k21> "87Sr 6733 AO 00:03" ("global virtual channels") refnum<k21> "87Sr 6733 AO 00:04" ("global virtual channels") refnum<k21> "87Sr 6733 AO 00:05" ("global virtual channels") refnum<k21> "87Sr 6733 AO 00:06" ("global virtual channels") refnum<k21> "87Sr 6733 AO 00:07" ("global virtual channels")] -> w551
        frame 0, Default {
          n104 = call "Display Message to User2"() -> ("Cancel"=w605:bool)  [unwired: 10 in, 1 out]
          n105 = Stop(stop? (T)=w605) -> ()
        }
        frame 1 {
        }
        frame 2 {
        }
        frame 3 {
        }
        frame 4 {
        }
        frame 5 {
        }
        frame 6 {
        }
        frame 7 {
        }
        frame 8 {
        }
      }
      n106 = property class="DAQmx Device"("Active Device"=tag "Dev1") -> ("Identification:Product Type"=w585:string)  [unwired: 2 in, 2 out]
      n107 = Equal?(x=w585, y="PCI-6733") -> (x = y?=w588:bool)
      n108 = case shown="True" w588 {
        tunnel: [w601 "PCI-6733 OK"] -> w587
        tunnel: "error in" -> [w602 w603]
        tunnel: [w600 w603] -> w583
        frame False {
          w601 = "PCI-6221 not found."
          n109 = Unbundle(w602) -> ()  [unwired: 3 out]
          n110 = Bundle(cluster=w602, "source"=w601) -> (w600:errorcluster)  [unwired: 2 in]
        }
        frame True {
        }
      }
      "6733 Status" <- w587
      n111 = case shown="True" "Case Constant\n(See Context Help) 3" {
        tunnel: w580 -> [_ w594]
        tunnel: w581 -> [_ w593]
        tunnel: w583 -> [w591 w592]
        tunnel: [w591 w592] -> w552
        frame False {
        }
        frame True {
          # "Clears tasks _before_ writing new waveform.\nError is not hooked up so that program will finish\nrunning either way."
          n112 = call <vilib>:"DAQmx Stop Task.vi"("task/channels in"=w593) -> ("task out"=w598:refnum<k21>, "error out"=w599:errorcluster)  [unwired: 13 in]
          n113 = call <vilib>:"DAQmx Clear Task.vi"("task in"=w598, "error in"=w599) -> ("error out"=w595:errorcluster)  [unwired: 13 in]
          n114 = call <vilib>:"DAQmx Stop Task.vi"("task/channels in"=w594, "error in"=w595) -> ("task out"=w596:refnum<k21>, "error out"=w597:errorcluster)  [unwired: 12 in]
          n115 = call <vilib>:"DAQmx Clear Task.vi"("task in"=w596, "error in"=w597) -> ()  [unwired: 13 in, 1 out]
        }
      }
      n116 = call <vilib>:"DAQmx Create Task.vi"("new task name"="87Sr Red Waveform", "auto cleanup"=FALSE, "global virtual channels"=w551, "error in"=w552) -> ("task out"=w579:refnum<k21>, "error out"=w575:errorcluster)  [unwired: 10 in]
      n117 = call-poly <vilib>:"DAQmx Timing.vi"("task/channels in"=w579, "sample mode"=w545, "rate"=w543, "source"=tag "/Dev1/Ctr0InternalOutput", "error in"=w575) -> ("task out"=w578:refnum<k21>, "error out"=w574:errorcluster)  [unwired: 9 in]
      n118 = call-poly <vilib>:"DAQmx Write.vi"("task/channels in"=w578, "data"=w542, "timeout"=10.0, "error in"=w574) -> ("task out"=w577:refnum<k21>, "error out"=w553:errorcluster)  [unwired: 9 in, 1 out]
      n119 = call <vilib>:"DAQmx Create Task.vi"("new task name"="87Sr 6733 Counter Output", "auto cleanup"=FALSE, "error in"=w553) -> ("task out"=w566:refnum<k21>, "error out"=w565:errorcluster)  [unwired: 11 in]
      n120 = call-poly <vilib>:"DAQmx Create Virtual Channel.vi"("task in"=w566, "frequency"=w543, "counter"=tag "Dev1/ctr0", "error in"=w565, "idle state"=w556) -> ("task out"=w567:refnum<k21>, "error out"=w564:errorcluster)  [unwired: 9 in]
      n121 = call-poly <vilib>:"DAQmx Timing.vi"("task/channels in"=w567, "sample mode"=w557, "samples per channel"=w541, "error in"=w564) -> ("task out"=w568:refnum<k21>, "error out"=w563:errorcluster)  [unwired: 10 in]
      n122 = call-poly <vilib>:"DAQmx Trigger.vi"("task/channels in"=w568, "source"=tag "/Dev1/PFI6", "edge"=w546, "error in"=w563) -> ("task out"=w569:refnum<k21>, "error out"=w562:errorcluster)  [unwired: 10 in]
      n123 = property class="DAQmx Trigger"(reference=w569, error in=w562, "Start:More:Retriggerable"=TRUE) -> (reference out=w570:refnum<k21>, error out=w561:errorcluster)
      n124 = call <vilib>:"DAQmx Start Task.vi"("task/channels in"=w577, "error in"=w561) -> ("task out"=→"87Sr 6733 adiabatic loading task out":refnum<k21>, "error out"=w560:errorcluster)  [unwired: 12 in]
      n125 = call <vilib>:"DAQmx Start Task.vi"("task/channels in"=w570, "error in"=w560) -> ("task out"=→"87Sr 6733 counter task out":refnum<k21>, "error out"=→"error out":errorcluster)  [unwired: 12 in]
      n126 = call <vilib>:"Simple Error Handler.vi"("type of dialog (OK msg:1)"=w544) -> ()  [unwired: 4 in, 5 out]
      "wvfrm size" <- w541
    }
  }
